vi "day4_1.vi"() -> ()   [LabVIEW 2012]
panel:
  out "Iteration 2":i32
  out "Iteration 1":i32
  in  "stop":bool
  out "Waveform Chart 2":dbl(graph)
  out "Waveform Chart":dbl(graph)
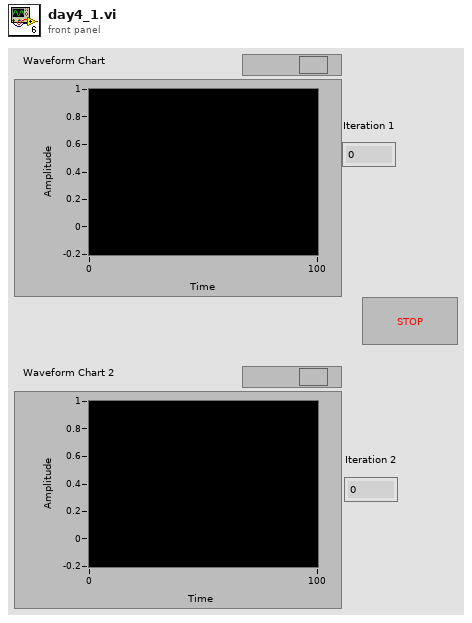
[diagram p1: front panel]
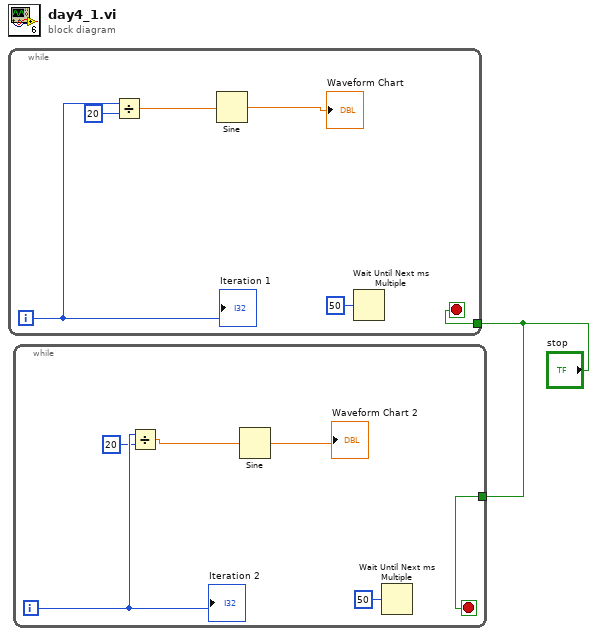
[diagram p0: block diagram]
diagram:
  n1 = while {
    tunnel: "stop" -> [w2]
    i -> [w3]
    stop <- w2 stop-if-true
    n2 = Divide(x=w3, y=20 ("x")) -> (x/y=w5:dbl)
    n3 = Sine(x=w5) -> (sin(x)=→"Waveform Chart":dbl)
    n4 = Wait Until Next ms Multiple(millisecond multiple=u32 50) -> ()  [unwired: 1 out]
    "Iteration 1" <- w3
  }
  n5 = while {
    tunnel: "stop" -> [w8]
    i -> [w10]
    stop <- w8 stop-if-true
    n6 = Divide(x=w10, y=20 ("x")) -> (x/y=w11:dbl)
    n7 = Sine(x=w11) -> (sin(x)=→"Waveform Chart 2":dbl)
    n8 = Wait Until Next ms Multiple(millisecond multiple=u32 50) -> ()  [unwired: 1 out]
    "Iteration 2" <- w10
  }
